vi "Build Channel Cluster Array.vi"() -> (3 "Channels out":cluster{"Channels":T1[]})   [LabVIEW 2023, in "Climate Chamber - 2 Channel.lvclass"]
uses:
  Climate Chamber - 2 Channel.lvclass
  Utilities/Channel.ctl
  Climate Chamber - 2 Channel.lvclass/Climate Chamber - 2 Channel.ctl
  Utilities/Utilities.lvlib
panel:
  in  "Chiller Cluster - 2 Channel.lvclass":refnum<class "Climate Chamber - 2 Channel.lvclass">
  in  "Channels in":cluster{"Channels":T1[]}
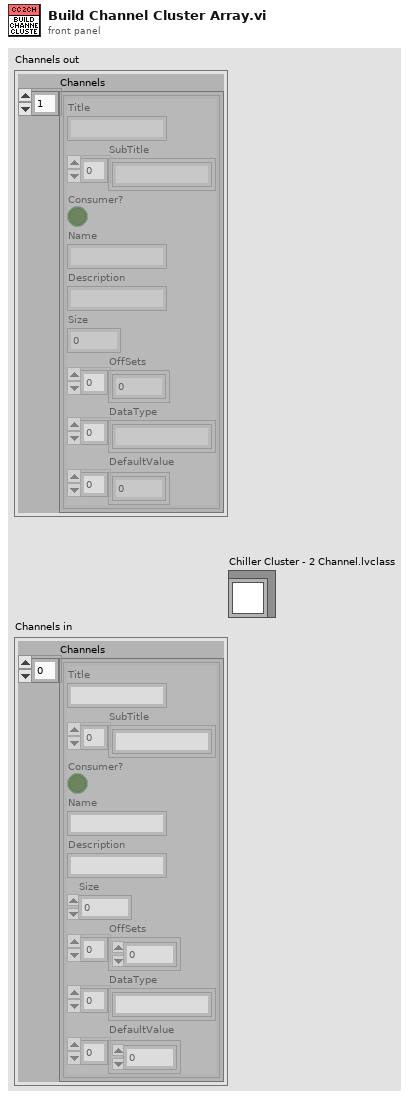
[diagram p1: front panel]
types:
  T1 = typedef "Utilities.lvlib/Channel.ctl" = cluster{"Title":string, "SubTitle":string[], "Consumer?":bool, "Name":string, "Description":string, "Size":i32, "OffSets":i32[], "DataType":string[], "DefaultValue":dbl[]}
  T2 = cluster{"OnOff.ACT":bool, "ErrorAcknowledge.ACT":bool}
  T3 = cluster{"OnOff.STS":i32, "Error.STS":i32, "Watchdog.STS":i32}
  T4 = cluster{"Temperature.ch01.SP":dbl, "TemperatureMIN.ch01.SP":dbl, "TemperatureMAX.ch01.SP":dbl, "TemperatureGrad.ch01.SP":dbl, "Humidity.ch01.SP":dbl, "HumidityMIN.ch01.SP":dbl, "HumidityMAX.ch01.SP":dbl, "HumidityGrad.ch01.SP":dbl}
  T5 = cluster{"Temperature.ch01.AV":dbl, "Humidity.ch01.AV":dbl}
  T6 = cluster{"Temperature.ch02.SP":dbl, "TemperatureMIN.ch02.SP":dbl, "TemperatureMAX.ch02.SP":dbl, "TemperatureGrad.ch02.SP":dbl, "Humidity.ch02.SP":dbl, "HumidityMIN.ch02.SP":dbl, "HumidityMAX.ch02.SP":dbl, "HumidityGrad.ch02.SP":dbl}
  T7 = cluster{"Temperature.ch02.AV":dbl, "Humidity.ch02.AV":dbl}
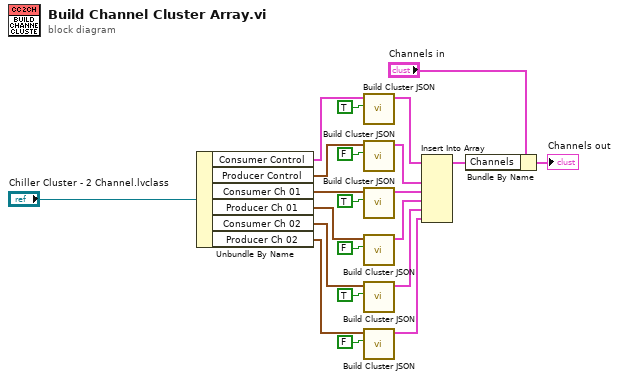
[diagram p0: block diagram]
diagram:
  n1 = Unbundle By Name("Chiller Cluster - 2 Channel.lvclass") -> ("Consumer Control"=w22:T2, "Producer Control"=w21:T3, "Consumer Ch 01"=w10:T4, "Producer Ch 01"=w11:T5, "Consumer Ch 02"=w2:T6, "Producer Ch 02"=w1:T7)
  n2 = call "Build Cluster JSON.vi"("Consumer?"=TRUE, "Cluster"=w22) -> ("Array"=w18:T1[])  [unwired: 9 in]
  n3 = call "Build Cluster JSON.vi"("Consumer?"=FALSE, "Cluster"=w21) -> ("Array"=w17:T1[])  [unwired: 9 in]
  n4 = call "Build Cluster JSON.vi"("Consumer?"=TRUE, "Cluster"=w10) -> ("Array"=w9:T1[])  [unwired: 9 in]
  n5 = call "Build Cluster JSON.vi"("Consumer?"=FALSE, "Cluster"=w11) -> ("Array"=w8:T1[])  [unwired: 9 in]
  n6 = call "Build Cluster JSON.vi"("Consumer?"=TRUE, "Cluster"=w2) -> ("Array"=w4:T1[])  [unwired: 9 in]
  n7 = call "Build Cluster JSON.vi"("Consumer?"=FALSE, "Cluster"=w1) -> ("Array"=w3:T1[])  [unwired: 9 in]
  n8 = Insert Into Array(array=w18, new element #1=w17, new element #2=w9, new element #3=w8, new element #4=w4, new element #5=w3) -> (w15:T1[])  [unwired: 1 in]
  n9 = Bundle By Name(cluster="Channels in", "Channels"=w15) -> (→"Channels out":cluster{"Channels":T1[]})
